vi "Toggle.vi"(8 "error in (no error)":errorcluster, 10 "Dirrection":enum16{"Forward", "Reverse"}(ring), 11 "State in":refnum<class "Parent Actor.lvclass">) -> (0 "error out":errorcluster, 3 "State out":refnum<class "Parent Actor.lvclass">)   [LabVIEW 2015, in "Parent Actor.lvclass"]
uses:
  Parent Actor.lvclass
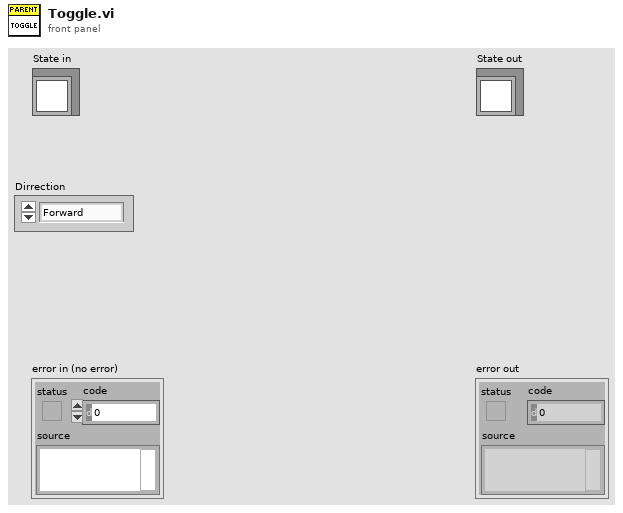
[diagram p1: front panel]
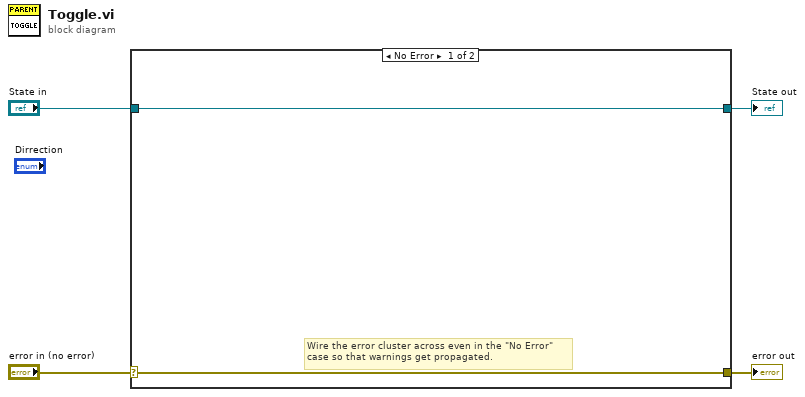
[diagram p0: block diagram]
diagram:
  n1 = case shown="No Error" "error in (no error)" {
    selector: "error in (no error)" -> [w5 w8]
    tunnel: [w5 w8] -> w3
    tunnel: [w6 w7] -> w1
    tunnel: "State in" -> [w6 w7]
    frame No Error {
      # "Wire the error cluster across even in the \"No Error\"\ncase so that warnings get propagated."
    }
    frame Error {
    }
  }
  "error out" <- w3
  "State out" <- w1
